vi "Get Tags from String.vi"(8 "error in (no error)":errorcluster, 11 "Input String":string) -> (0 "error out":errorcluster, 3 "Tags[]":string[](array[string]))   [LabVIEW 2016, in "SLL String.lvlib"]
doc: "Searches and returns the list of tags present in a string. Tags are expected to be in the format [Tag]"
uses:
  SLL String.lvlib
  <vilib>/regexp/Match Regular Expression.xnode
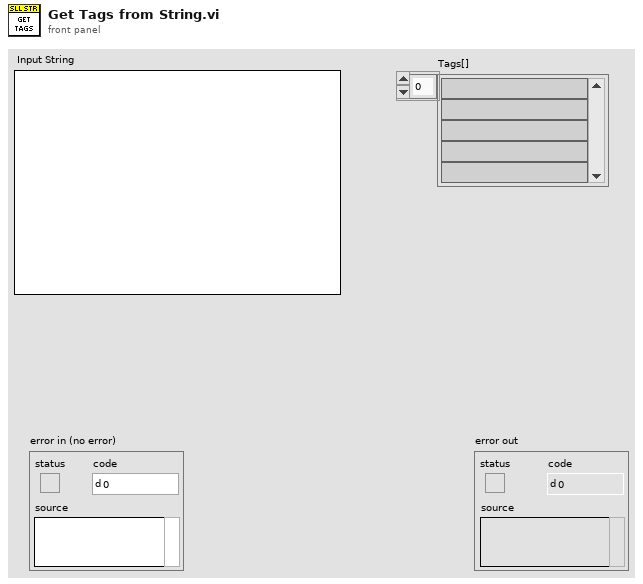
[diagram p1: front panel]
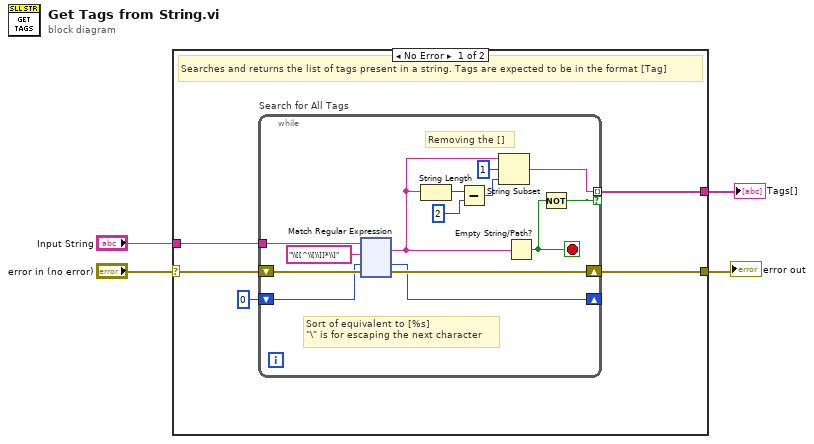
[diagram p0: block diagram]
diagram:
  n1 = case shown="No Error" "error in (no error)" {
    selector: "error in (no error)" -> [w8 w138]
    tunnel: "Input String" -> [w9 _]
    tunnel: [w7 w138] -> w1
    tunnel: [w5 _] -> w2
    frame No Error {
      # "Searches and returns the list of tags present in a string. Tags are expected to be in the format [Tag]"
      n2 = while "Search for All Tags" {
        tunnel: w9 -> [w23]
        shift-right: [w21] -> w7
        shift-left: w8 -> [w22]
        shift-right: [w19] -> _
        shift-left: 0 ("offset past match") -> [w18]
        tunnel: [w15] -> w5 mode=indexing if=w16
        stop <- w17 stop-if-true
        # "Removing the []"
        # "Sort of equivalent to [%s]\n\"\\\" is for escaping the next character"
        n3 = xnode "Match Regular Expression"("input string"=w23, "regular expression"="\\[[^\\[\\]]*\\]", "offset (0)"=w18, "error in"=w22) -> ("whole match"=w13:string, "offset past match"=w19:i32, "error out"=w21:errorcluster)  [unwired: 2 in, 2 out]
        n4 = String Length(string=w13) -> (length=w12:i32)
        n5 = Subtract(x=w12, y=2) -> (x-y=w10:i32)
        n6 = String Subset(string=w13, offset (0)=1, length (rest)=w10) -> (substring=w15:string)
        n7 = Empty String/Path?(string/path=w13) -> (empty?=w17:bool)
        n8 = Not(x=w17) -> (.not. x?=w16:bool)
      }
    }
    frame Error {
    }
  }
  "error out" <- w1
  "Tags[]" <- w2
